vi "generate step function.vi"(6 "sampling info":cluster{"Fs":dbl, "#s":dbl}={"Fs"=1000.0, "#s"=1000.0} {"Fs" format="%.2p"}, 7 "N_fast":dbl, 8 "error in (no error)":errorcluster, 9 "Offset_slow":dbl, 10 "N_slow":dbl, 11 "step_size":dbl) -> (0 "error out":errorcluster, 2 "Waveform_slow":waveform(dbl))   [LabVIEW 2012, in "ImagingModeSPIM.lvclass"]
uses:
  ImagingModeSPIM.lvclass
panel:
  out "Waveform Graph":dbl[](graph)
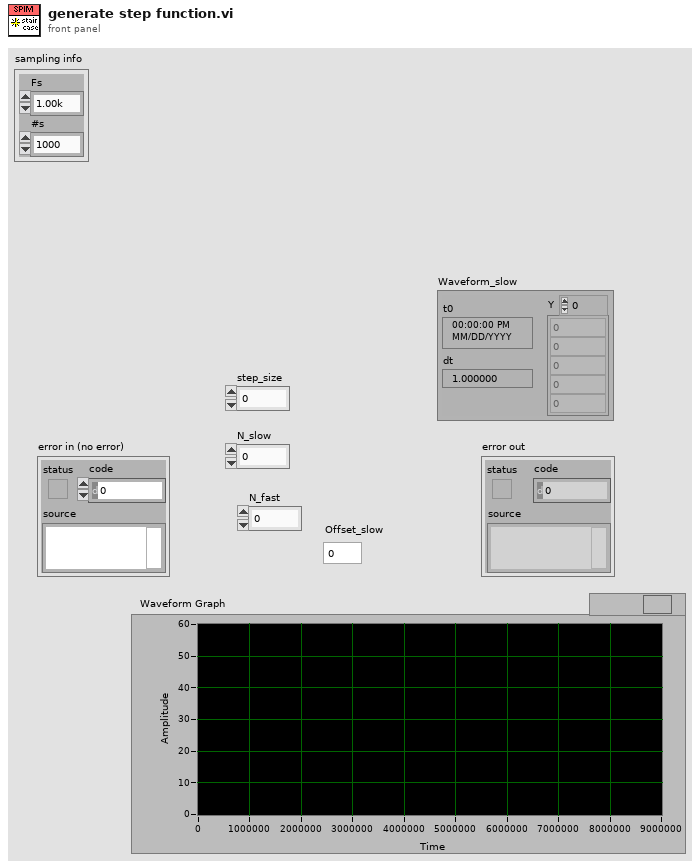
[diagram p1: front panel]
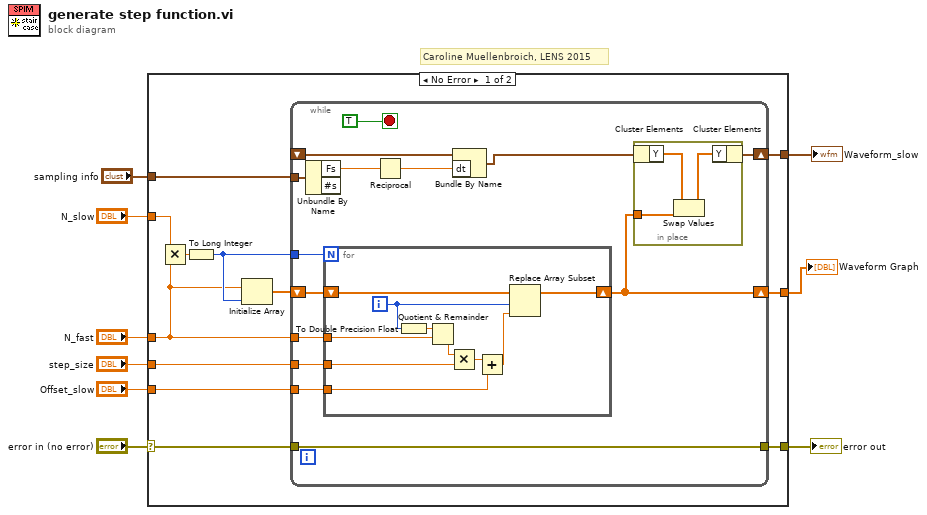
[diagram p0: block diagram]
diagram:
  # "Caroline Muellenbroich, LENS 2015"
  n1 = case shown="No Error" "error in (no error)" {
    selector: "error in (no error)" -> [w20 w49]
    tunnel: [w19 w49] -> w8
    tunnel: "N_slow" -> [w14 _]
    tunnel: "step_size" -> [w18 _]
    tunnel: [w21 _] -> w5
    tunnel: "N_fast" -> [w11 _]
    tunnel: "Offset_slow" -> [w17 _]
    tunnel: "sampling info" -> [w16 _]
    tunnel: [w10 _] -> w1
    frame No Error {
      n2 = Multiply(x=w14, y=w11) -> (x*y=w15:dbl)
      n3 = To Long Integer(number=w15) -> (32bit integer=w12:i32)
      n4 = Initialize Array(w11, w12) -> (w13:dbl[])
      n5 = while {
        tunnel: w20 -> [w35]
        tunnel: [w35] -> w19
        shift-right: [w32] -> w21
        shift-left: _ -> [w31]
        tunnel: w11 -> [w27]
        tunnel: w18 -> [w30]
        tunnel: w17 -> [w29]
        tunnel: w16 -> [w28]
        tunnel: w12 -> [w24]
        shift-right: [w22] -> w10
        shift-left: w13 -> [w23]
        stop <- TRUE ("stop") stop-if-true
        n6 = Unbundle By Name(w28) -> ("Fs"=w26:dbl)  [unwired: 1 out]
        n7 = for {
          N: w24 -> [_]
          tunnel: w27 -> [w45]
          tunnel: w30 -> [w42]
          tunnel: w29 -> [w41]
          shift-right: [w39] -> w22
          shift-left: w23 -> [w38]
          i -> [w36]
          n8 = To Double Precision Float(number=w36) -> (double precision float=w44:dbl)
          n9 = Quotient & Remainder(x=w44, y=w45) -> (floor(x/y)=w43:dbl)  [unwired: 1 out]
          n10 = Multiply(x=w43, y=w42) -> (x*y=w40:dbl)
          n11 = Add(x=w40, y=w41) -> (x+y=w37:dbl)
          n12 = Replace Array Subset(array=w38, new element=w37, index=w36) -> (w39:dbl[])
        }
        n13 = Reciprocal(x=w26) -> (1/x=w25:dbl)
        n14 = Bundle By Name(cluster=w31, "dt"=w25) -> (w33:waveform(dbl))
        n15 = in-place {
          in-place-border: w22 -> [w46]
          n16 = in-place-cluster #1(w33) -> ("Y"=w48:dbl[])
          n17 = Swap Values(12:w48, 14:w46) -> (1:w47:dbl[])  [unwired: 1 in, 1 out]
          n18 = in-place-cluster #1("Y"=w47) -> (w32:waveform(dbl))
        }
      }
    }
    frame Error {
    }
  }
  "error out" <- w8
  "Waveform_slow" <- w5
  "Waveform Graph" <- w1
